vi "SectorBiopsy.vi"() -> ()   [LabVIEW 2022 SP3]
uses:
  <vilib>/Utility/file.llb/Read From Spreadsheet File (DBL).vi
  <vilib>/Analysis/NI_AALBase.lvlib
  <vilib>/Analysis/baseanly.llb/Mean (DBL).vi
panel:
  out "Current File":string
  out "Avf Pwr Spectrum":T1(graph)
  out "length y (mm)":dbl format="%.3f"
  out "length x (mm)":dbl format="%.3f"
  out "inc y (mm)":dbl format="%.3f"
  out "inc x (mm)":dbl format="%.3f"
  in  "cal file options":u16(ring)=3 items=["Use Header Info (B&K)", "Use Header Info (Hit)", "Specify Header Values (B&K)", "Specify Header Values (Hit)", "Specify Header, no Cal file"]
  in  "Save to Spectra.txt?":bool
  out "Mean params values":T2 {"pts in fit" format="%.2f"; "midband fit" format="%.2f"; "intercept (b)" format="%.2f"; "slope (m)" format="%.2f"}
  in  "Ring":u16(ring) items=["Select Files in Listbox", "Choose list of file", "Biopsy location list"]
  in  "Use Selected Files":bool
  in  "Choose Directory":path
  in  "Listbox":i32[](listbox)=[0]
  out "raw data":dbl[][](graph)
  out "Cal File Att":string
  out "RF File Att":string
  in  "FFT size":u16(ring)=6 items=["next 2^n", "8", "16", "32", "64", "128", "256", "512"]
  in  "Cal File Name":string
  in  "Fit band":T3={"start"=3.5, "stop freq"=8.0, "center freq"=5.75} {"center freq" format="%.2f"; "stop freq" format="%.2f"; "start" format="%.2f"}
  out "current file path":path
  # "Spectrum Fit Parameters"
  # "This program uses a 64 pt sliding window to find the average parameter values of the boxed region. If a calibration file is used, select either B&K or Hitachi format. The Hitachi file is a cross calibration file and needs to be a two column, tab dilineated text file. First column midband, second intercept.  Cross calibration should be the same values as those used by Spectrasonics but may need need to be formatted. 2.5 dB correction included in B&K option but not in Hitachi because it is part of the cross calibration"
  # "Defaults"
  # "448 62\n448 241\n459 62\n459 241"
  # "Green left bottom, red right top, yellow right bottom. Green & red same x value, green & yellow same y value."
  # "© 2000-2010 Riverside Research Institute"
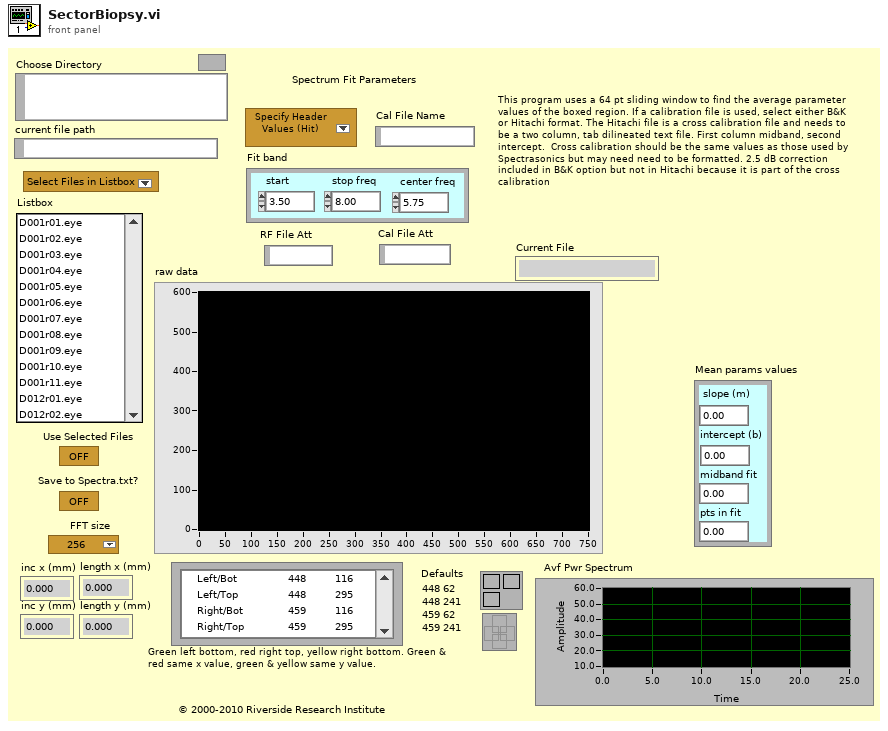
[diagram p1: front panel]
types:
  T1 = cluster{"fo of fit":dbl, "df (MHz)":dbl, "power spectrum in dB":dbl[]}
  T2 = cluster{"slope (m)":dbl, "intercept (b)":dbl, "midband fit":dbl, "pts in fit":dbl}
  T3 = cluster{"start":dbl, "stop freq":dbl, "center freq":dbl}
  T4 = cluster{"x1":dbl, "y1":dbl, "x2":dbl, "y2":dbl, "x3":dbl, "y3":dbl, "y3 2":dbl, "x3 2":dbl}
  T5 = cluster{"Cursor.Cursor X":dbl, "Cursor.Cursor Y":dbl, "Cursor.Cursor X":dbl, "Cursor.Cursor Y":dbl, "Cursor.Cursor X":dbl, "Cursor.Cursor Y":dbl, "Cursor.Cursor X":dbl, "Cursor.Cursor Y":dbl}
  T6 = cluster{"x1":dbl, "y1":dbl, "x2":dbl, "y2":dbl, "x3":dbl, "y3":dbl, "y3 2":dbl, "x3 2":dbl}[]
  T7 = cluster{"x1":dbl, "y1":dbl, "x2":dbl, "y2":dbl, "x3":dbl, "y3":dbl, "x4":dbl, "y4":dbl}[]
  T8 = cluster{"TPI start":dbl[], "#TPI pts":dbl[], "Subset TPI offset":dbl}
  T9 = cluster{"x start":i32, "x length":i32, "y start":i32, "y length":i32}
  T10 = cluster{"X right":dbl, "X left":dbl, "Y low":dbl, "Y high":dbl}
  T11 = typedef "Header.ctl" = cluster{"header info":cluster{"Header":string, "Head length":i16}, "A/D info":cluster{"# rf points per line":u16, "# lines per scan":u16, "sample rate MHz":u16, "# A/D bits":i16, "# bytes per A/D":u16, "TGC Flag":u16, "A/D Type":string}, "Tranducer Info":cluster{"bandwidth":sgl, "center freq":sgl, "start freq":sgl, "ID":i32}, "Scan Info":cluster{"delay":sgl, "pivot distance":sgl, "sector scan angle":sgl, "operator":string, "Scan Mode":string, "location":string}, "Time/Date Info":cluster{"date":string, "time":string}, "RF Info":cluster{"RF file name":string, "RF file att":string, "RF cal file name":string, "RF cal file att":string}, "Patient Info":cluster{"ID":string, "extended ID":string, "age":u16, "sex":string, "previously\nscanned":string, "PSA":sgl, "LOS":u8, "Ethnicty 2":u8, "Race":u8}, "Tissue Type":cluster{"organ":i16, "disease type":i16, "disease location":i16}, "Votage scaling":cluster{"Digitizer (dB)":sgl, "Gain (dB)":sgl, "Atten (dB)":sgl}, "Comment":string, "Misc Info":cluster{"avg num":i16, "c speed":i16, "Div By or SF zones":i16, "XMIT CHS":u8, "RCV CHS":u8}, "Therapy Parameters":cluster{"Theraputic Freq (MHz)":sgl, "Time on (s)":sgl, "Therapy amplitude (mV)":sgl, "Lines Before":u16, "Lines After":u16}, "Scan Settings":cluster{"Energy (uJ or V)":u8, "Damp (Ohm) or Fc":u8, "HP Filt (KHz)":u8, "LP Filt (MHz)":u8, "Gain (db)":u8, "prf (kHz)":sgl, "Distance between\nscan lines (mm)":u16, "Distance between\nscan planes (mm)":u16}, "Compression Parameters":cluster{"F1 (MHz)":sgl, "F2 (MHz)":sgl, "% taper":sgl, "duration":sgl}, "Patient Info Xtra":cluster{"First Name":string, "Last Name":string, "Notes":string}}
  T12 = cluster{"RF file name":string, "RF file att":string, "RF cal file name":string, "RF cal file att":string}
  T13 = cluster{"start freq":sgl, sgl, "center freq":sgl}
  T14 = cluster{"RF cal file name":string, "RF file att":string, "Cal File Name":string, "RF cal file att":string}
  T15 = cluster{"slope (m)":dbl[][], "intercept (b)":dbl[][], "midband fit":dbl[][], "pts in fit":dbl}
  T16 = cluster{"slope (m)":dbl, "m stand dev":dbl, "intercept (b)":dbl, "b stand dev":dbl, "MSE":dbl, "midband fit":dbl, "pts in fit":dbl}
  T17 = cluster{"fo of fit":dbl, "df (MHz)":dbl, dbl[]}[]
  T18 = cluster{"[0]":dbl, "[1]":dbl, "[2]":dbl, "number of pts":dbl}
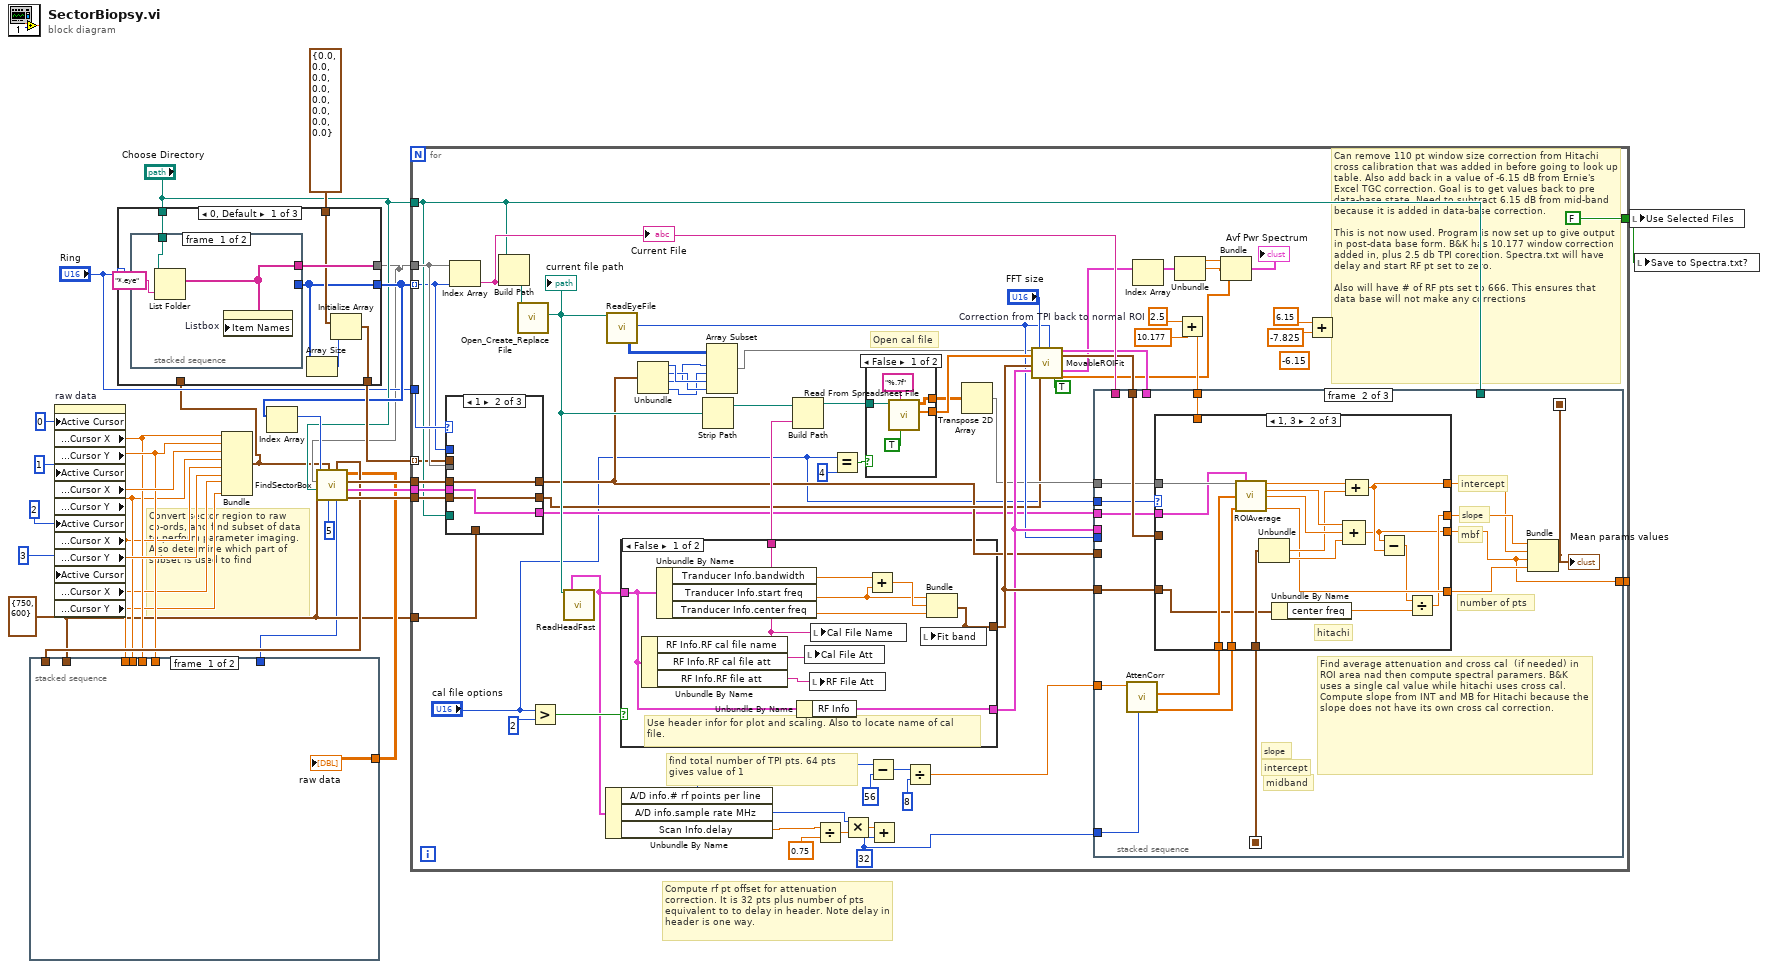
[diagram p0: block diagram]
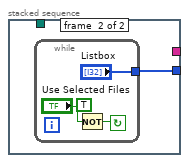
[diagram p2: hidden frame]
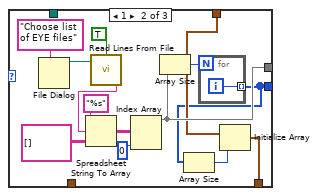
[diagram p3: hidden frame]
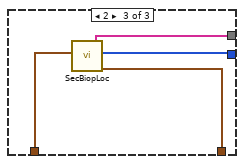
[diagram p4: hidden frame]
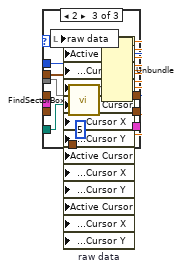
[diagram p6: hidden frame]
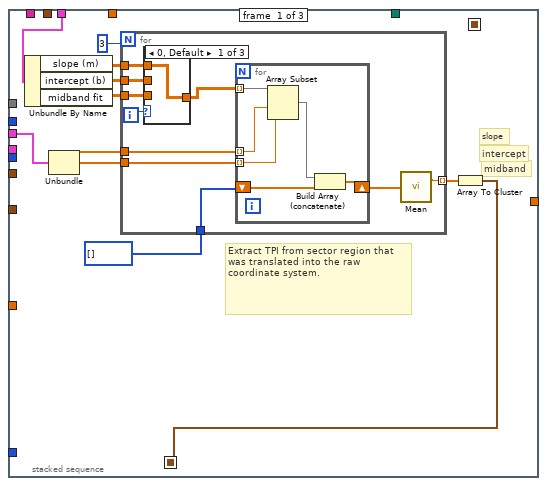
[diagram p7: hidden frame]
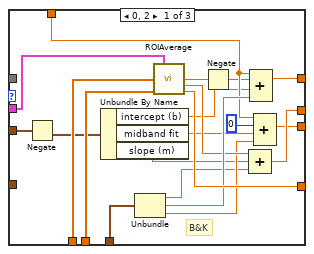
[diagram p10: hidden frame]
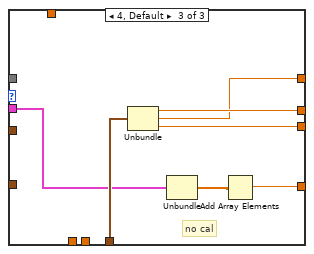
[diagram p11: hidden frame]
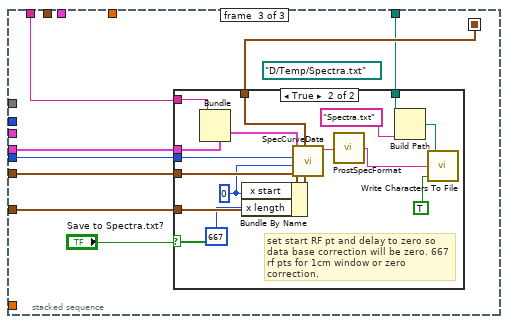
[diagram p12: hidden frame]
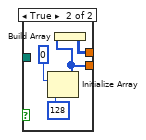
[diagram p14: hidden frame]
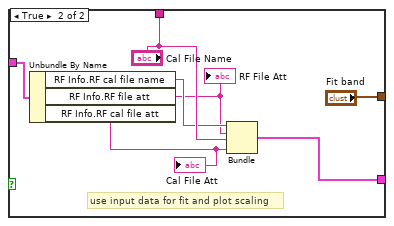
[diagram p15: hidden frame]
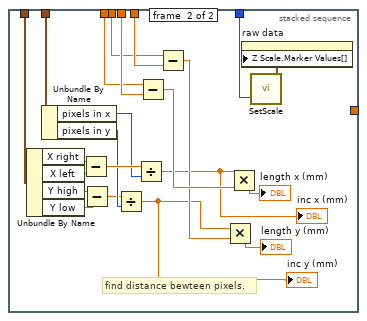
[diagram p16: hidden frame]
diagram:
  w14 = cluster{"pixels in x":i16, "pixels in y":i16} {"pixels in x"=750, "pixels in y"=600} ("sector size")
  # "Compute rf pt offset for attenuation correction. It is 32 pts plus number of pts equivalent to to delay in header. Note delay in header is one way."
  # "Convert sector region to raw co-ords, and find subset of data to perform parameter imaging. Also determine which part of subset is used to find"
  n1 = property on="raw data" class="IntGraph (strict)"("Active Cursor"=0, "Active Cursor"=1, "Active Cursor"=2, "Active Cursor"=3) -> ("Cursor.Cursor Position:Cursor X"=w19:dbl, "Cursor.Cursor Position:Cursor Y"=w20:dbl, "Cursor.Cursor Position:Cursor X"=w27:dbl, "Cursor.Cursor Position:Cursor Y"=w18:dbl, "Cursor.Cursor Position:Cursor X"=w17:dbl, "Cursor.Cursor Position:Cursor Y"=w26:dbl, "Cursor.Cursor Position:Cursor X"=w8:dbl, "Cursor.Cursor Position:Cursor Y"=w7:dbl)  [unwired: 2 in, 2 out]
  n2 = Bundle("Cursor.Cursor X"=w19, "Cursor.Cursor Y"=w20, "Cursor.Cursor X"=w27, "Cursor.Cursor Y"=w18, "Cursor.Cursor X"=w17, "Cursor.Cursor Y"=w26, "Cursor.Cursor X"=w8, "Cursor.Cursor Y"=w7) -> (w1:T5)  [unwired: 1 out]
  n3 = case shown="0, Default" "Ring" {
    tunnel: [w35 w48 w60] -> w2
    tunnel: "Choose Directory" -> [w34 _ _]
    tunnel: [w31 w44 w61] -> w11
    tunnel: w1 -> [_ _ w59]
    tunnel: [w32 w43 w58] -> w13
    tunnel: T4 {"x1"=0.0, "y1"=0.0, "x2"=0.0, "y2"=0.0, "x3"=0.0, "y3"=0.0, "y3 2"=0.0, "x3 2"=0.0} ("Sector EndPts") -> [w33 w45 _]
    frame 0, Default {
      n4 = stacked-sequence {
        tunnel: [w37 _] -> w35
        tunnel: w34 -> [w36 _]
        tunnel: [_ w39] -> w31
        frame #0 {
          n5 = List Folder(path=w36, pattern="*.eye") -> (filenames=w37:string[])  [unwired: 1 in, 4 out]
          n6 = property on="Listbox" class="LstBox (strict)"("Item Names"=w37) -> ()  [unwired: 2 in, 2 out]
        }
        frame #1 {
          n7 = while {
            tunnel: ["Listbox"] -> w39
            stop <- w41 continue-if-true
            (unwired) TRUE
            n8 = Not(x="Use Selected Files") -> (.not. x?=w41:bool)
          }
        }
      }
      n9 = Array Size(array=w31) -> (size(s)=w30:i32)
      n10 = Initialize Array(w33, w30) -> (w32:T6)
    }
    frame 1 {
      n11 = File Dialog(7:"Choose list of EYE files" ("prompt")) -> (3:w54:path)  [unwired: 1 in, 8 out]
      n12 = call <vilib>:"Read Lines From File.vi"("convert eol? (no:F)"=TRUE, "file path (dialog if empty)"=w54) -> ("line string"=w49:string)  [unwired: 1 in, 6 out]
      n13 = Spreadsheet String To Array(format string="%s", spreadsheet string=w49, array type (2D Dbl)=string[][] [] ("Array Constant")) -> (array=w53:string[][])  [unwired: 1 in]
      n14 = Index Array(array=w53, index (col)=0) -> (element=w48:string[])  [unwired: 1 in]
      n15 = Array Size(array=w48) -> (size(s)=w47:i32)
      n16 = for {
        N: w47 -> [_]
        tunnel: [w57] -> w44 mode=indexing
        i -> [w57]
      }
      n17 = Array Size(array=w44) -> (size(s)=w46:i32)
      n18 = Initialize Array(w45, w46) -> (w43:T6)
    }
    frame 2 {
      n19 = call "SecBiopLoc.vi"("Ref Sector EndPts"=w59) -> ("Sector Endpts out"=w58:T7, "Listbox"=w61:i32[], "File names"=w60:string[])  [unwired: 1 in, 3 out]
    }
  }
  n20 = Index Array(array=w11) -> (element=w10:i32)  [unwired: 1 in]
  n21 = call "FindSectorBox.vi"("reduce pts by factor of"=5, "Sector EndPts"=w1, "sector size"=w14, "directory path"="Choose Directory", "File Array"=w2, "File Index"=w10) -> ("Fit Array"=w23:cluster{i32, i32, dbl, i32}, "ROI (PramImage Subset co-ords)"=w22:T8, "Subset dimensions"=w24:T9, "raw sector out"=w16:dbl[][], "A/D bits"=w3:u16, "Axis scaling Params"=w21:T10)
  n22 = stacked-sequence {
    tunnel: w3 -> [_ w64]
    tunnel: w21 -> [_ w84]
    tunnel: w14 -> [_ w82]
    tunnel: w16 -> [w62 _]
    tunnel: w20 -> [_ w74]
    tunnel: w19 -> [_ w73]
    tunnel: w18 -> [_ w72]
    tunnel: w17 -> [_ w71]
    frame #0 {
      "raw data" <- w62
    }
    frame #1 {
      # "find distance bewteen pixels."
      n23 = Unbundle By Name(w84) -> ("X right"=w78:dbl, "X left"=w76:dbl, "Y high"=w75:dbl, "Y low"=w77:dbl)
      n24 = Unbundle By Name(w82) -> ("pixels in x"=w81:i16, "pixels in y"=w80:i16)
      n25 = Subtract(x=w78, y=w76) -> (x-y=w83:dbl)
      n26 = Subtract(x=w75, y=w77) -> (x-y=w79:dbl)
      n27 = Divide(x=w79, y=w80) -> (x/y=w68:dbl)
      "inc y (mm)" <- w68
      n28 = Divide(x=w83, y=w81) -> (x/y=w67:dbl)
      "inc x (mm)" <- w67
      n29 = Subtract(x=w71, y=w73) -> (x-y=w70:dbl)
      n30 = Subtract(x=w72, y=w74) -> (x-y=w69:dbl)
      n31 = Multiply(x=w68, y=w69) -> (x*y=→"length y (mm)":dbl)
      n32 = Multiply(x=w67, y=w70) -> (x*y=→"length x (mm)":dbl)
      n33 = call "SetScale.vi"("# A/D bits"=w64) -> ("Array"=w63:cluster{dbl, u32}[])  [unwired: 1 in]
      n34 = property on="raw data" class="IntGraph (strict)"("Z Scale.Marker Values[]"=w63) -> ()  [unwired: 2 in, 2 out]
    }
  }
  n35 = for {
    tunnel: w2 -> [w109]
    tunnel: "Choose Directory" -> [w108]
    tunnel: w11 -> [w106] mode=indexing
    tunnel: w23 -> [w111]
    tunnel: w24 -> [w113]
    tunnel: w22 -> [w112]
    tunnel: [FALSE] -> w15
    tunnel: "Ring" -> [w114]
    tunnel: w14 -> [w110]
    tunnel: w13 -> [w107] mode=indexing
    tunnel: [w87] -> _
    (unwired) -6.15
    w115 = 32
    w118 = 2.5  # Correction from TPI back to normal ROI
    # "Can remove 110 pt window size correction from Hitachi cross calibration that was added in before going to look up table. Also add back in a value of -6.15 dB from Ernie's Excel TGC correction. Goal is to get values back to pre data-base state. Need to subtract 6.15 dB from mid-band because it is added in data-base correction.\n\nThis is not now used. Program is now set up to give output in post-data base form. B&K has 10.177 window correction added in, plus 2.5 db TPI corection. Spectra.txt will have delay and start RF pt set to zero.\n\nAlso will have # of RF pts set to 666. This ensures that data base will not make any corrections"
    # "find total number of TPI pts. 64 pts gives value of 1"
    # "Open cal file"
    n36 = case shown="1" w114 {
      tunnel: [w151 w154 w176] -> w96
      tunnel: w113 -> [w151 w154 _]
      tunnel: [w150 w153 w175] -> w95
      tunnel: w112 -> [w150 w153 _]
      tunnel: [w149 w152 w174] -> w97
      tunnel: w111 -> [w149 w152 _]
      tunnel: w110 -> [_ _ w173]
      tunnel: w109 -> [_ _ w172]
      tunnel: w108 -> [_ _ w170]
      tunnel: w107 -> [_ _ w169]
      tunnel: w106 -> [_ _ w158]
      frame 0, Default {
      }
      frame 1 {
      }
      frame 2 {
        n37 = call "FindSectorBox.vi"("reduce pts by factor of"=5, "Sector EndPts"=w169, "sector size"=w173, "directory path"=w170, "File Array"=w172, "File Index"=w158) -> ("Fit Array"=w174:cluster{i32, i32, dbl, i32}, "ROI (PramImage Subset co-ords)"=w175:T8, "Subset dimensions"=w176:T9, "raw sector out"=w159:dbl[][])  [unwired: 2 out]
        n38 = local write "raw data"(w159) -> ()
        n39 = Unbundle(w169) -> ("x1"=w165:dbl, "y1"=w164:dbl, "x2"=w163:dbl, "y2"=w162:dbl, "x3"=w161:dbl, "y3"=w160:dbl, "x4"=w156:dbl, "y4"=w155:dbl)
        n40 = property on="raw data" class="IntGraph (strict)"("Active Cursor"=0, "Cursor.Cursor Position:Cursor X"=w165, "Cursor.Cursor Position:Cursor Y"=w164, "Active Cursor"=1, "Cursor.Cursor Position:Cursor X"=w163, "Cursor.Cursor Position:Cursor Y"=w162, "Active Cursor"=2, "Cursor.Cursor Position:Cursor X"=w161, "Cursor.Cursor Position:Cursor Y"=w160, "Active Cursor"=3, "Cursor.Cursor Position:Cursor X"=w156, "Cursor.Cursor Position:Cursor Y"=w155) -> ()  [unwired: 2 in, 2 out]
      }
    }
    n41 = Index Array(array=w109, index=w106) -> (element=w127:string)
    "Current File" <- w127
    n42 = Build Path(base path=w108, name or relative path=w127) -> (appended path=w143:path)
    n43 = call <vilib>:"Open_Create_Replace File.vi"("file path"=w143) -> ("new file path"=w142:path)  [unwired: 5 in, 5 out]
    "current file path" <- w142
    n44 = Greater?(x="cal file options", y=2) -> (0:w136:bool)
    n45 = call "ReadHeadFast.vi"("new file path"=w142) -> ("Header In"=w86:T11)  [unwired: 15 in, 3 out]
    n46 = Unbundle By Name(w86) -> ("A/D info.# rf points per line"=w122:u16, "A/D info.sample rate MHz"=w123:u16, "Scan Info.delay"=w85:sgl)
    n47 = call "ReadEyeFile.vi"("new file path"=w142) -> ("2-D data array"=w90:i16[][], "sample rate MHz"=w139:u16)  [unwired: 1 in, 16 out]
    n48 = case shown="False" w136 {
      tunnel: w86 -> [w302 w311]
      tunnel: [w308 "Fit band"] -> w141
      tunnel: [w304 "Cal File Name"] -> w146
      tunnel: [w301 w314] -> w140
      frame False {
        # "Use header infor for plot and scaling. Also to locate name of cal\nfile."
        n49 = Unbundle By Name(w302) -> ("RF Info.RF cal file name"=w304:string, "RF Info.RF cal file att"=w305:string, "RF Info.RF file att"=w303:string)
        n50 = Unbundle By Name(w302) -> ("Tranducer Info.bandwidth"=w310:sgl, "Tranducer Info.start freq"=w306:sgl, "Tranducer Info.center freq"=w309:sgl)
        n51 = Unbundle By Name(w302) -> ("RF Info"=w301:T12)
        n52 = local write "Cal File Att"(w305) -> ()
        n53 = local write "RF File Att"(w303) -> ()
        n54 = local write "Cal File Name"(w304) -> ()
        n55 = Add(x=w310, y=w306) -> (x+y=w307:sgl)
        n56 = Bundle("start freq"=w306, w307, "center freq"=w309) -> (w308:T13)  [unwired: 1 out]
        n57 = local write "Fit band"(w308) -> ()
      }
      frame True {
        # "use input data for fit and plot scaling"
        n58 = Unbundle By Name(w311) -> ("RF Info.RF cal file name"=w315:string, "RF Info.RF file att"=w312:string, "RF Info.RF cal file att"=w313:string)
        "RF File Att" <- w312
        "Cal File Att" <- w313
        n59 = Bundle("RF cal file name"=w315, "RF file att"=w312, "Cal File Name"="Cal File Name", "RF cal file att"=w313) -> (w314:T14)  [unwired: 1 out]
      }
    }
    n60 = Unbundle(w96) -> ("x start"=w94:i32, "x length"=w93:i32, "y start"=w92:i32, "y length"=w91:i32)
    n61 = Strip Path(path=w142) -> (stripped path=w144:path)  [unwired: 1 out]
    n62 = Array Subset(array=w90, index (row)=w92, length (row)=w91, index (col)=w94, length (col)=w93) -> (w89:i16[][])
    n63 = Build Path(base path=w144, name or relative path=w146) -> (appended path=w137:path)
    n64 = Divide(x=w85, y=0.75) -> (x/y=w125:dbl)
    n65 = Equal?(x="cal file options", y=4) -> (x = y?=w135:bool)
    n66 = Multiply(x=w123, y=w125) -> (x*y=w124:dbl)
    n67 = case shown="False" w135 {
      tunnel: w137 -> [w296 _]
      tunnel: [w293 w298] -> w148
      tunnel: [w292 w297] -> w133
      frame False {
        n68 = call-poly <vilib>:"Read From Spreadsheet File.vi"("transpose (no:F)"=TRUE, "format (%.3f)"="%.7f", "file path (dialog if empty)"=w296) -> ("first row"=w293:dbl[], "all rows"=w292:dbl[][])  [unwired: 1 in, 6 out]
      }
      frame True {
        n69 = Initialize Array(0, 128) -> (w298:i32[])
        n70 = Build Array(w298) -> (w297:i32[][])
      }
    }
    n71 = Subtract(x=w122, y=56) -> (x-y=w130:i32)
    n72 = Add(x=w124, y=w115) -> ()  [unwired: 1 out]
    n73 = Divide(x=w130, y=8) -> (x/y=w119:dbl)
    n74 = Transpose 2D Array(2D array=w133) -> (transposed array=w132:dbl[][])
    n75 = call "MovableROIFit.vi"("input array"=w89, "calibration data"=w148, "Fit band"=w141, "RF Info"=w140, "FFT size for"="FFT size", "Fit array"=w97, "freq (MHz)"=w139, "convert output to dB?"=TRUE) -> ("Raw Fit Data"=w105:T15, "Cal params"=w104:T16, "Plots"=w102:T17, "power spectrum in dB"=w100:dbl[])  [unwired: 5 in, 3 out]
    n76 = Index Array(array=w102) -> (element=w103:cluster{"fo of fit":dbl, "df (MHz)":dbl, dbl[]})  [unwired: 1 in]
    n77 = Unbundle(w103) -> ("fo of fit"=w98:dbl, "df (MHz)"=w101:dbl)  [unwired: 1 out]
    n78 = Add(x=w118, y=10.177) -> (x+y=w116:dbl)
    n79 = stacked-sequence {
      seq-local: [_ w207 _] -> [_ _ w273]
      seq-local: [w177 _ _] -> [_ w214 _]
      tunnel: w141 -> [_ w209 w275]
      tunnel: w140 -> [_ _ w269]
      tunnel: w139 -> [_ _ w274]
      tunnel: w96 -> [_ _ w270]
      tunnel: w105 -> [w187 _ _]
      tunnel: w104 -> [_ w222 _]
      tunnel: "cal file options" -> [_ w221 _]
      tunnel: w95 -> [w182 w215 _]
      tunnel: w132 -> [_ w220 _]
      tunnel: w108 -> [_ _ w272]
      tunnel: w127 -> [_ _ w268]
      tunnel: w119 -> [_ w218 _]
      tunnel: w115 -> [_ w219 _]
      tunnel: w116 -> [_ w210 _]
      tunnel: [_ w208 _] -> w87
      frame #0 {
        # "midband"
        # "intercept"
        # "slope"
        # "Extract TPI from sector region that was translated into the raw coordinate system."
        n80 = Unbundle By Name(w187) -> ("slope (m)"=w185:dbl[][], "intercept (b)"=w184:dbl[][], "midband fit"=w183:dbl[][])
        n81 = Unbundle(w182) -> ("TPI start"=w180:dbl[], "#TPI pts"=w181:dbl[])  [unwired: 1 out]
        n82 = for {
          N: 3 -> [_]
          tunnel: w185 -> [w196]
          tunnel: w184 -> [w195]
          tunnel: w183 -> [w194]
          tunnel: [w193] -> w178 mode=indexing
          tunnel: w180 -> [w192]
          tunnel: w181 -> [w191]
          tunnel: i32[] [] ("Array Constant") -> [w189]
          i -> [w197]
          n83 = case shown="0, Default" w197 {
            tunnel: [w198 w199 w200] -> w188
            tunnel: w196 -> [w198 _ _]
            tunnel: w195 -> [_ w199 _]
            tunnel: w194 -> [_ _ w200]
            frame 0, Default {
            }
            frame 1 {
            }
            frame 2 {
            }
          }
          n84 = for {
            tunnel: w188 -> [w206] mode=indexing
            tunnel: w191 -> [w205] mode=indexing
            tunnel: w192 -> [w204] mode=indexing
            shift-right: [w203] -> w190
            shift-left: w189 -> [w202]
            n85 = Array Subset(array=w206, index=w204, length=w205) -> (w201:dbl[])
            n86 = Build Array (concatenate)(w201, w202) -> (w203:dbl[])
          }
          n87 = call-poly <vilib>:"Mean.vi"("X"=w190) -> ("mean"=w193:dbl)  [unwired: 1 out]
        }
        n88 = Array To Cluster(array=w178) -> (cluster=w177:cluster{"[0]":dbl, "[1]":dbl, "[2]":dbl})
      }
      frame #1 {
        # "slope"
        # "intercept"
        # "midband"
        # "slope"
        # "mbf"
        # "intercept"
        # "number of pts"
        # "Find average attenuation and cross cal  (if needed) in ROI area nad then compute spectral paramers. B&K uses a single cal value while hitachi uses cross cal. Compute slope from INT and MB for Hitachi because the slope does not have its own cross cal correction."
        n89 = call "AttenCorr.vi"("Offset"=w219, "ROIs in x"=w218) -> ("slope correction"=w216:dbl[], "midband correction"=w217:dbl[])  [unwired: 5 in, 2 out]
        n90 = case shown="1, 3" w221 {
          tunnel: w222 -> [w243 _ _]
          tunnel: w220 -> [_ w260 _]
          tunnel: w215 -> [w242 w259 w263]
          tunnel: w217 -> [w228 w258 _]
          tunnel: w216 -> [w241 w257 _]
          tunnel: w214 -> [w238 w255 w267]
          tunnel: [w231 w246 w266] -> w213
          tunnel: [w232 w245 w265] -> w212
          tunnel: [w230 w244 w264] -> w208
          tunnel: [w240 w250 w261] -> w211
          tunnel: w210 -> [w233 _ _]
          tunnel: w209 -> [_ w248 _]
          frame 0, 2 {
            # "B&K"
            n91 = Negate(x=w243) -> (-x=w227:T16)
            n92 = Unbundle By Name(w227) -> ("intercept (b)"=w226:dbl, "midband fit"=w225:dbl, "slope (m)"=w224:dbl)
            n93 = Unbundle(w238) -> ("[0]"=w223:dbl, "[1]"=w237:dbl, "[2]"=w234:dbl)
            n94 = call "ROIAverage.vi"("ROI (PramImage Subset co-ords)"=w242, "midband att"=w228, "slope att"=w241) -> ("av att mb"=w239:dbl, "av att slope"=w236:dbl, "number of pts"=w240:dbl)  [unwired: 1 in, 9 out]
            n95 = Negate(x=w239) -> (-x=w229:dbl)
            n96 = Compound Arithmetic op=ADD(w236, w224, w223) -> (w231:dbl)
            n97 = Compound Arithmetic op=ADD(w233, w229, w226, w237) -> (w232:dbl)
            n98 = Compound Arithmetic op=ADD(w233, 0, w225, w234) -> (w230:dbl)
          }
          frame 1, 3 {
            # "hitachi"
            n99 = call "ROIAverage.vi"("Hitachi Cal"=w260, "ROI (PramImage Subset co-ords)"=w259, "midband att"=w258, "slope att"=w257) -> ("av cal int"=w256:dbl, "av cal mb"=w253:dbl, "av att mb"=w254:dbl, "number of pts"=w250:dbl)  [unwired: 8 out]
            n100 = Unbundle(w255) -> ("[1]"=w251:dbl, "[2]"=w252:dbl)  [unwired: 1 out]
            n101 = Unbundle By Name(w248) -> ("center freq"=w247:dbl)
            n102 = Compound Arithmetic op=ADD(w253, w254, w252) -> (w244:dbl)
            n103 = Compound Arithmetic op=ADD(w256, w251) -> (w245:dbl)
            n104 = Subtract(x=w244, y=w245) -> (x-y=w249:dbl)
            n105 = Divide(x=w249, y=w247) -> (x/y=w246:dbl)
          }
          frame 4, Default {
            # "no cal"
            n106 = Unbundle(w267) -> ("[0]"=w266:dbl, "[1]"=w265:dbl, "[2]"=w264:dbl)
            n107 = Unbundle(w263) -> ("#TPI pts"=w262:dbl[])  [unwired: 2 out]
            n108 = Add Array Elements(numeric array=w262) -> (sum=w261:dbl)
          }
        }
        n109 = Bundle("[0]"=w213, "[1]"=w212, "[2]"=w208, "number of pts"=w211) -> (w207:T18)  [unwired: 1 out]
        "Mean params values" <- w207
      }
      frame #2 {
        (unwired) path "D:/Temp/Spectra.txt"
        n110 = case shown="True" "Save to Spectra.txt?" {
          tunnel: w275 -> [_ w280]
          tunnel: w269 -> [_ w282]
          tunnel: w270 -> [_ w279]
          tunnel: w274 -> [_ w291]
          tunnel: w273 -> [_ w284]
          tunnel: w272 -> [_ w287]
          tunnel: w268 -> [_ w283]
          frame False {
          }
          frame True {
            w277 = 0
            # "set start RF pt and delay to zero so data base correction will be zero. 667 rf pts for 1cm window or zero correction."
            n111 = Bundle(cluster=w282, "RF cal file name"=w283) -> (w281:T14)  [unwired: 3 out]
            n112 = Bundle By Name(cluster=w279, "x start"=w277, "x length"=667) -> (w278:T9)
            n113 = call "SpecCurveData.vi"("Fit band"=w280, "Fit params"=w284, "Array Subset"=w278, "delay"=w277, "sample rate MHz"=w291, "RF Info"=w281) -> ("Spectra data"=w290:string)  [unwired: 1 in, 4 out]
            n114 = call "ProstSpecFormat.vi"("Spectra.txt old (string)"=w290) -> ("Spectra.txt new out"=w288:string)
            n115 = Build Path(base path=w287, name or relative path="Spectra.txt") -> (appended path=w285:path)
            n116 = call <vilib>:"Write Characters To File.vi"("append to file? (new file:F)"=TRUE, "character string"=w288, "file path (dialog if empty)"=w285) -> ()  [unwired: 3 out]
          }
        }
      }
    }
    n117 = Bundle("fo of fit"=w98, "df (MHz)"=w101, "power spectrum in dB"=w100) -> (→"Avf Pwr Spectrum":T1)  [unwired: 1 out]
    n118 = Add(x=6.15, y=-7.825) -> ()  [unwired: 1 out]
  }
  n119 = local write "Use Selected Files"(w15) -> ()
  n120 = local write "Save to Spectra.txt?"(w15) -> ()
